vi "Init Msg Default.vi"() -> (2 "Msg":refnum<class "Msg.lvclass">)   [LabVIEW 2020, in "jettl.lvlib" / "Start jettl Msg.lvlib" / "Start Msg.lvlib"]
doc: "jettl 6.14.1.98\nNathan Davis - Nathan Davis\nCopyright (c) 2026, Nathan Davis\nMIT"
uses:
  Start Msg.lvlib
  Msg/Msg.lvclass
  Start Msg/Start Msg.lvclass
  C:/git/jettl/src/jettl/jettl/Msg/Msg.lvclass
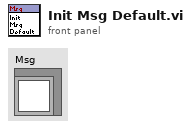
[diagram p1: front panel]
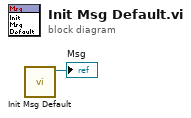
[diagram p0: block diagram]
diagram:
  n1 = call "Init Msg Default.vi"() -> ("Start Msg out"=→"Msg":refnum<class "Start Msg.lvclass">)  [unwired: 11 in]
